vi "init.vi"(8 "error in (no error)":errorcluster, 11 "FlukeDMM in":refnum<class "FlukeDMM.lvclass">) -> (0 "error out":errorcluster, 3 "FlukeDMM out":refnum<class "FlukeDMM.lvclass">)   [LabVIEW 2013, in "FlukeDMM.lvlib" / "FlukeDMM.lvclass"]
uses:
  <userlib>/Common/Devices/FlukeDMM/FlukeDMM/FlukeDMM.lvclass
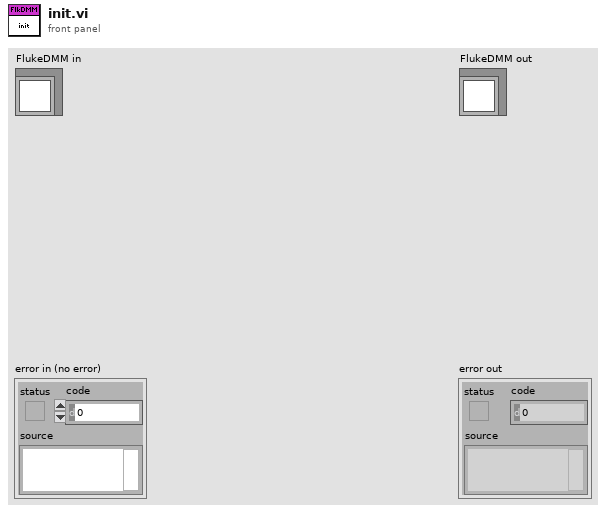
[diagram p1: front panel]
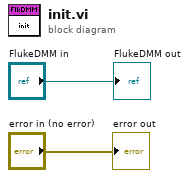
[diagram p0: block diagram]
diagram:
  "error out" <- "error in (no error)"
  "FlukeDMM out" <- "FlukeDMM in"
